vi "Test_PublicationLocked_RequestLock_ErrorReturned.vi"(8 "error in (no error)":errorcluster, 11 "TestMediator In":refnum<class "TestMediator.lvclass">) -> (0 "error out":errorcluster, 3 "TestMediator Out":refnum<class "TestMediator.lvclass">)   [LabVIEW 2017, in "TestMediator.lvclass"]
uses:
  TestMediator.lvclass
  Mediator/Mediator.lvclass
  C:/Program Files (x86)/National Instruments/LabVIEW 2017/vi.lib/ActorFramework/Actor/Actor.lvclass
  Transport/QueueTransport/QueueTransport.lvclass/QueueTransport.ctl
  IMediator/IMediator Messages/Lock Publication Msg/Lock Publication Msg.lvclass/Lock Publication Msg.ctl
  <vilib>/ActorFramework/Message Enqueuer/Message Enqueuer.lvclass/Message Enqueuer.ctl
  <vilib>/ActorFramework/Message Enqueuer/Enqueue.vi
  Transport/QueueTransport/QueueTransport.lvclass
  C:/Git/mva-framework/Framework/IMediator/ITransport/ITransport.lvclass
  IMediator/IMediator Messages/Lock Publication Msg/Lock Publication Msg.lvclass
  C:/Program Files (x86)/National Instruments/LabVIEW 2017/vi.lib/ActorFramework/Message/Message.lvclass
  <vilib>/ActorFramework/Stop Msg/Stop Msg.lvclass
  <vilib>/Utility/error.llb/Error Cluster From Error Code.vi
  <vilib>/ActorFramework/Message Priority Queue/Priority Enqueue.vi
  IMediator/IPublicationPolicy/IPublicationPolicy.lvclass
  IMediator/ITransport/ITransport.lvclass
  <vilib>/addons/_JKI Toolkits/VI Tester/TestCase.llb/TestCase.lvclass
  <vilib>/ActorFramework/Actor/Actor.lvclass
  C:/Program Files (x86)/National Instruments/LabVIEW 2017/vi.lib/addons/_JKI Toolkits/VI Tester/TestCase.llb/TestCase.lvclass
panel:
  out "Lock Return Error":errorcluster
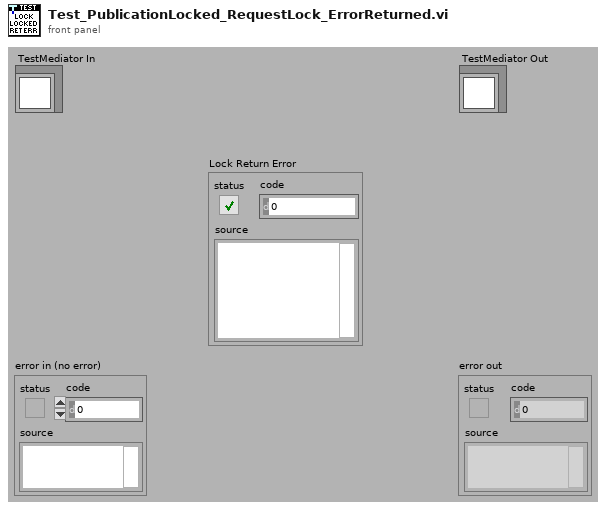
[diagram p1: front panel]
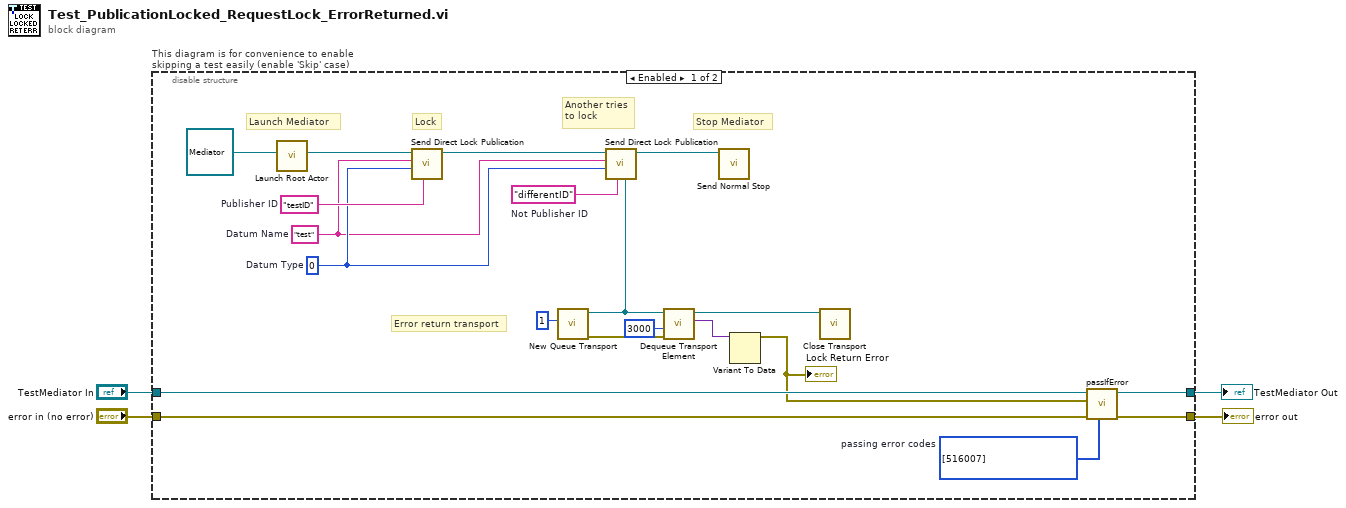
[diagram p0: block diagram]
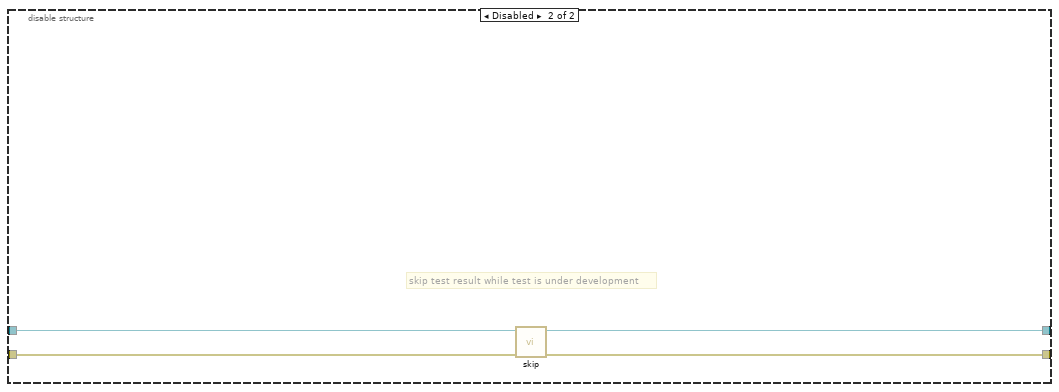
[diagram p2: hidden frame]
diagram:
  n1 = disable-structure "This diagram is for convenience to enable skipping a test easily (enable 'Skip' case)" shown="Enabled" {
    disable-tunnel: "TestMediator In" -> [w24 w28]
    disable-tunnel: [w23 w26] -> w1
    disable-tunnel: [w22 w27] -> w3
    disable-tunnel: "error in (no error)" -> [w21 w25]
    frame Enabled {
      w5 = i32[] [516007]  # passing error codes
      w11 = "differentID"  # Not Publisher ID
      w14 = "testID"  # Publisher ID
      w13 = 0  # Datum Type
      w12 = "test"  # Datum Name
      # "Error return transport"
      # "Lock"
      # "Launch Mediator"
      # "Stop Mediator"
      # "Another tries\nto lock"
      n2 = call <vilib>:"Launch Root Actor.vi"("Actor"=refnum<class "Mediator.lvclass"> refnum ("Mediator.lvlib:Mediator.lvclass")) -> ("Actor's Enqueuer"=w19:refnum<class "Message Enqueuer.lvclass">)  [unwired: 9 in, 1 out]
      n3 = call "Send Direct Lock Publication.vi"("Publisher ID"=w14, "Datum Type"=w13, "Datum Name"=w12, "Mediator Enqeuer"=w19) -> ("Mediator Enqueuer out"=w15:refnum<class "Message Enqueuer.lvclass">)  [unwired: 6 in, 1 out]
      n4 = call "New Queue Transport.vi"("Max Queue Size (-1)"=1) -> ("error out"=w9:errorcluster, "QueueTransport"=w8:refnum<class "QueueTransport.lvclass">)  [unwired: 9 in]
      n5 = call "Send Direct Lock Publication.vi"("Return Error Transport"=w8, "Publisher ID"=w11, "Datum Type"=w13, "Datum Name"=w12, "Mediator Enqeuer"=w15) -> ("Mediator Enqueuer out"=w10:refnum<class "Message Enqueuer.lvclass">)  [unwired: 5 in, 1 out]
      n6 = call "Dequeue Transport Element.vi"("error in (no error)"=w9, "Timeout In ms (-1)"=3000, "QueueTransport in"=w8) -> ("Data"=w6:variant, "QueueTransport out"=w16:refnum<class "QueueTransport.lvclass">)  [unwired: 5 in, 2 out]
      n7 = call <vilib>:"Send Normal Stop.vi"("Message Enqueuer"=w10) -> ()  [unwired: 10 in, 1 out]
      n8 = Variant To Data(Variant=w6) -> (data=w7:errorcluster)  [unwired: 2 in, 1 out]
      "Lock Return Error" <- w7
      n9 = call-dynamic "Close Transport.vi"("QueueTransport in"=w16) -> ()  [unwired: 10 in, 1 out]
      n10 = call-dynamic "passIfError.vi"("passing error codes (default = any error code)"=w5, "error in (no error)"=w21, "error"=w7, "TestCase in"=w24) -> ("error out"=w22:errorcluster, "TestCase out"=w23:refnum<class "TestMediator.lvclass">)  [unwired: 6 in]
    }
    frame Disabled {
      # "skip test result while test is under development"
      n11 = call <vilib>:"skip.vi"("error in (no error)"=w25, "TestCase in"=w28) -> ("error out"=w27:errorcluster, "TestCase out"=w26:refnum<class "TestMediator.lvclass">)  [unwired: 8 in]
    }
  }
  "error out" <- w3
  "TestMediator Out" <- w1
